vi "Scan Engine Update Slot Subpanel.vi"(7 "SubPanel Event":refnum<user-event>, 8 "error in (no error)":errorcluster, 9 "SubPanel Ref":refnum<vi>, 10 "RSI Module in":refnum<class "RSI Module.lvclass">, 11 "Node Ptr In":T1 format="%.0x") -> (0 "error out":errorcluster, 2 "RSI Module out":refnum<class "RSI Module.lvclass">, 3 "Node Ptr Out":T1 format="%.0x")   [LabVIEW 2017, in "Scan Engine Custom Device.lvlib"]
uses:
  Scan Engine Custom Device.lvlib
  <vilib>/NI Veristand/Custom Device API/Custom Device Item Ref.ctl
  Modules.lvlibp/RSI Module/RSI Module.lvclass
  Modules.lvlibp/RSI Module/SubPanel Command.ctl
  <vilib>/Utility/miscctls.llb/LVRectTypeDef.ctl
  Globals/SubPanel Controls.vi
  <vilib>/NI Veristand/Custom Device API/Custom Device API.lvlib
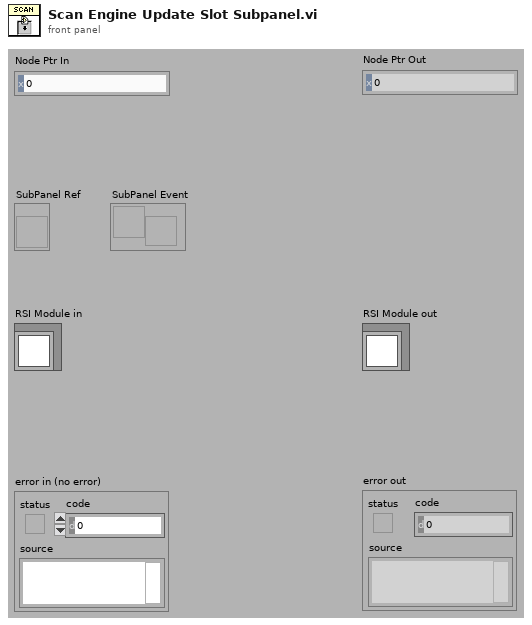
[diagram p1: front panel]
types:
  T1 = typedef "Custom Device API.lvlib/Custom Device Item Ref.ctl" = u64
  T2 = typedef "LVRectTypeDef.ctl" = cluster{"Left":i16, "Top":i16, "Right":i16, "Bottom":i16}
  T3 = typedef "LVBoundsTypeDef.ctl" = cluster{"Width":u32, "Height":u32}
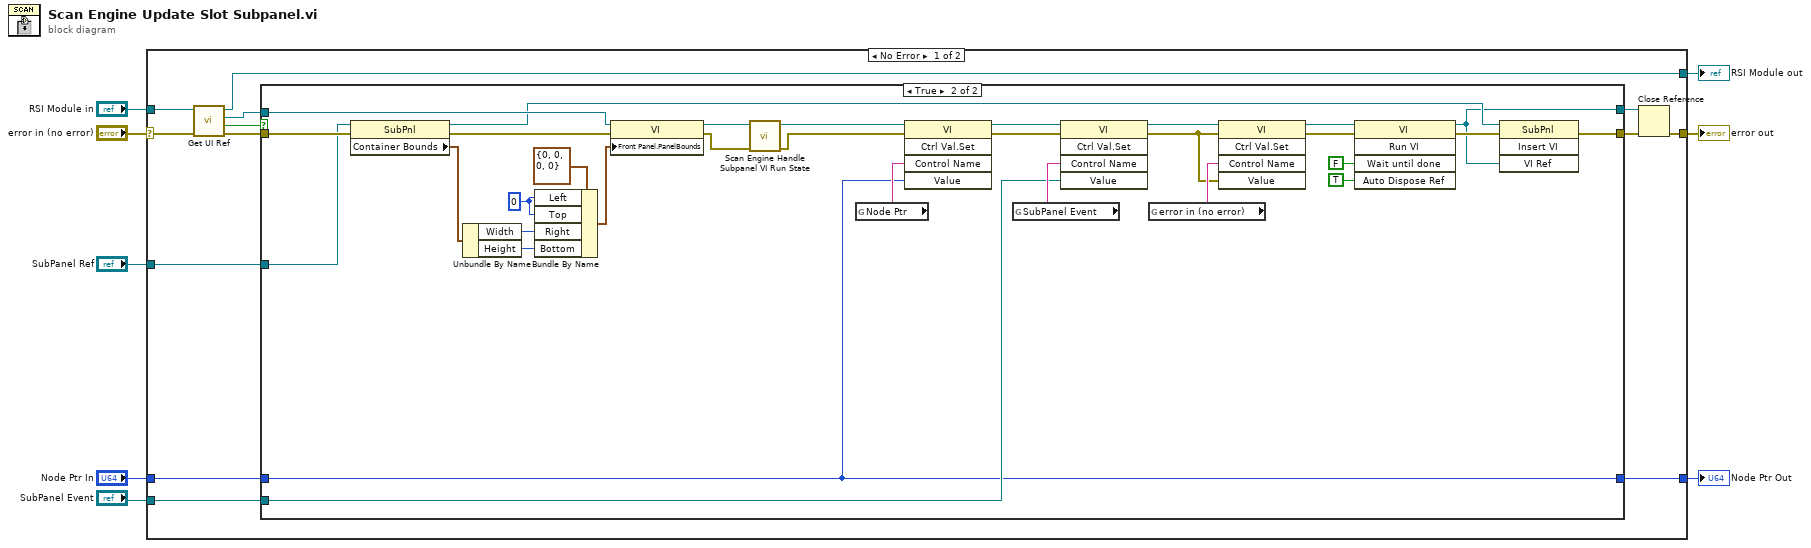
[diagram p0: block diagram]
diagram:
  n1 = case shown="No Error" "error in (no error)" {
    selector: "error in (no error)" -> [w11 w58]
    tunnel: "SubPanel Ref" -> [w21 _]
    tunnel: [w17 w58] -> w7
    tunnel: "Node Ptr In" -> [w16 w57]
    tunnel: "SubPanel Event" -> [w14 _]
    tunnel: "RSI Module in" -> [w13 w56]
    tunnel: [w12 w56] -> w4
    tunnel: [w9 w57] -> w2
    frame No Error {
      n2 = call-dynamic "Get UI Ref.vi"("error in (no error)"=w11, "RSI Module in"=w13) -> ("error out"=w15:errorcluster, "Show SubPanel?"=w10:bool, "VI Refnum"=w20:refnum<vi>, "RSI Module out"=w12:refnum<class "RSI Module.lvclass">)  [unwired: 6 in]
      n3 = case shown="True" w10 {
        tunnel: w21 -> [_ w35]
        tunnel: w20 -> [w23 w50]
        tunnel: [w23 w29] -> w19
        tunnel: [w24 w30] -> w18
        tunnel: w16 -> [w22 w36]
        tunnel: w15 -> [w24 w40]
        tunnel: w14 -> [_ w37]
        tunnel: [w22 w36] -> w9
        frame False {
        }
        frame True {
          w53 = i16 0 ("Left")
          n4 = property class="SubPnl"(reference=w35, error in=w40) -> (reference out=w32:refnum<vi>, error out=w39:errorcluster, "Container Bounds"=w51:T3)
          n5 = Unbundle By Name(w51) -> ("Width"=w54:u32, "Height"=w55:u32)
          n6 = Bundle By Name(cluster=T2 {"Left"=0, "Top"=0, "Right"=0, "Bottom"=0} ("Front Panel Window:Panel Bounds"), "Left"=w53, "Top"=w53, "Right"=w54, "Bottom"=w55) -> (w49:T2)
          n7 = property class="VI"(reference=w50, error in=w39, "Front Panel.PanelBounds"=w49) -> (reference out=w28:refnum<vi>, error out=w27:errorcluster)
          n8 = call "Scan Engine Handle Subpanel VI Run State.vi"("error in (no error)"=w27, "VI in"=w28) -> ("error out"=w26:errorcluster, "VI out"=w25:refnum<vi>)  [unwired: 8 in]
          n9 = global read "SubPanel Controls.vi" "Node Ptr"() -> (w41:string)
          n10 = invoke class="VI" method="Ctrl Val.Set"(reference=w25, error in=w26, "Control Name"=w41, "Value"=w36) -> (reference out=w48:refnum<vi>, error out=w47:errorcluster)  [unwired: 1 in, 3 out]
          n11 = global read "SubPanel Controls.vi" "SubPanel Event"() -> (w38:string)
          n12 = invoke class="VI" method="Ctrl Val.Set"(reference=w48, error in=w47, "Control Name"=w38, "Value"=w37) -> (reference out=w34:refnum<vi>, error out=w33:errorcluster)  [unwired: 1 in, 3 out]
          n13 = global read "SubPanel Controls.vi" "error in (no error)"() -> (w42:string)
          n14 = invoke class="VI" method="Ctrl Val.Set"(reference=w34, error in=w33, "Control Name"=w42, "Value"=w33) -> (reference out=w46:refnum<vi>, error out=w45:errorcluster)  [unwired: 1 in, 3 out]
          n15 = invoke class="VI" method="Run VI"(reference=w46, error in=w45, "Wait until done"=FALSE ("Wait Until Done"), "Auto Dispose Ref"=TRUE ("Auto Dispose Reference")) -> (reference out=w29:refnum<vi>, error out=w31:errorcluster)  [unwired: 1 in, 3 out]
          n16 = invoke class="SubPnl" method="Insert VI"(reference=w32, error in=w31, "VI Ref"=w29) -> (error out=w30:errorcluster)  [unwired: 1 in, 3 out]
        }
      }
      n17 = Close Reference(reference=w19, error in (no error)=w18) -> (error out=w17:errorcluster)
    }
    frame Error {
    }
  }
  "error out" <- w7
  "Node Ptr Out" <- w2
  "RSI Module out" <- w4
